vi "rpopup.vi"() -> ()   [LabVIEW 2014]
doc: "Target VI used in conjunction with the asynchronous call examples."
uses:
  subVI/version.vi
panel:
  in  "닫기":bool
  out "?":string="\n"
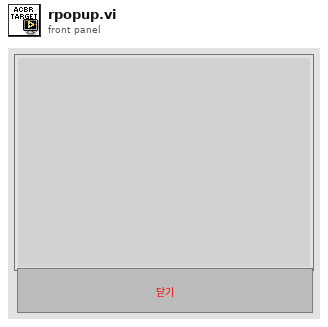
[diagram p1: front panel]
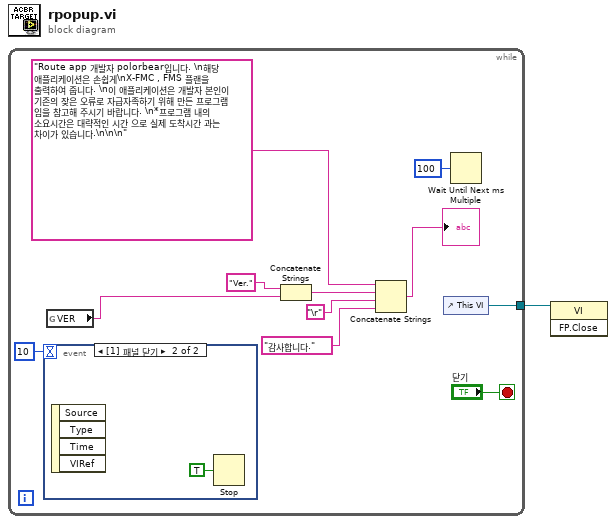
[diagram p0: block diagram]
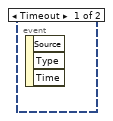
[diagram p2: hidden frame]
diagram:
  n1 = while {
    tunnel: [w11] -> w1
    stop <- "닫기" stop-if-true
    n2 = event shown="[1] 패널 닫기" {
      selector: _ -> [_ _]
      dyn-events: _ -> [_ _]
      timeout: 10 -> [_ _]
      event Timeout {
        n3 = event-data() -> ()  [unwired: 1 in, 3 out]
      }
      event Panel Close {
        n4 = event-data() -> ()  [unwired: 1 in, 4 out]
        n5 = Stop(stop? (T)=TRUE ("정지? (참)")) -> ()
      }
    }
    n6 = global read "version.vi" "VER"() -> (w6:string)
    n7 = Concatenate Strings("Ver." ("문자열"), w6) -> (w7:string)
    n8 = Concatenate Strings("Route app 개발자 polorbear입니다. \n해당 애플리케이션은 손쉽게\nX-FMC , FMS 플랜을 출력하여 줍니다. \n이 애플리케이션은 개발자 본인이 기존의 잦은 오류로 자급자족하기 위해 만든 프로그램 임을 참고해 주시기 바랍니다. \n*프로그램 내의 소요시간은 대략적인 시간 으로 실제 도착시간 과는 차이가 있습니다.\n\n\n", w7, "\r", "감사합니다." ("문자열")) -> (→"?":string)
    n9 = control-ref of="This VI"() -> (w11:refnum<vi>)
    n10 = Wait Until Next ms Multiple(millisecond multiple=u32 100 ("ms 배수")) -> ()  [unwired: 1 out]
  }
  n11 = invoke class="VI" method="FP.Close"(reference=w1) -> ()  [unwired: 2 in, 3 out]
